vi "ClusterwitharrayUNSETTYPE.vi"(1 "Cluster In":cluster{"Array In":void[]}) -> (0 "Cluster Out":cluster{"Array Out":void[]})   [LabVIEW 2011]
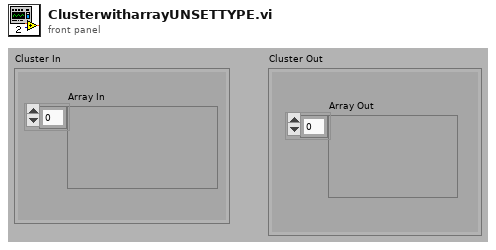
[diagram p1: front panel]
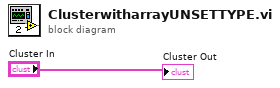
[diagram p0: block diagram]
diagram:
  "Cluster Out" <- "Cluster In"
